vi "calc_formula.vi"() -> ()   [LabVIEW 2021]
uses:
  <vilib>/gmath/NI_Gmath.lvlib
panel:
  out "status":bool
  in  "formula":string
  out "y value":dbl format="%0.2f"
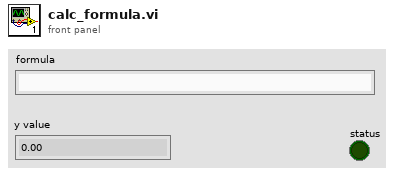
[diagram p1: front panel]
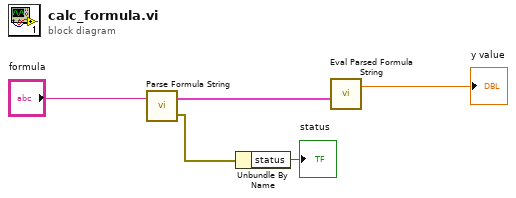
[diagram p0: block diagram]
diagram:
  n1 = call <vilib>:"Parse Formula String.vi"("formula"="formula") -> ("error out"=w2:errorcluster, "Parsed Formula"=w5:cluster{"Table":i32[][], "Y Values":dbl[]})  [unwired: 1 in]
  n2 = Unbundle By Name(w2) -> ("status"=→"status":bool)
  n3 = call <vilib>:"Eval Parsed Formula String.vi"("Parsed Formula"=w5) -> ("y value"=→"y value":dbl)  [unwired: 3 in, 1 out]
